vi "Init Error Logging.vi"(8 "error in (no error)":errorcluster, 11 "SOL-Server in":refnum<class "SOL-Server.lvclass">) -> (0 "error out":errorcluster, 3 "SOL-Server out":refnum<class "SOL-Server.lvclass">)   [LabVIEW 2020, in "Summer of LabVIEW.lvlib" / "SOL-Server.lvclass"]
uses:
  SOL-Server.lvclass
  SOL-Server.lvclass/SOL-Server.ctl
  Error Log.ctl
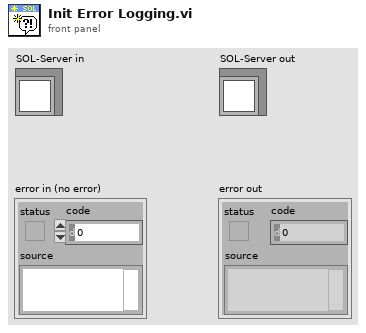
[diagram p1: front panel]
types:
  T1 = typedef "Summer of LabVIEW.lvlib/SOL-Server.lvclass/Error Log.ctl" = cluster{"Time Stamp":timestamp, "Code":i32, "Source":string}
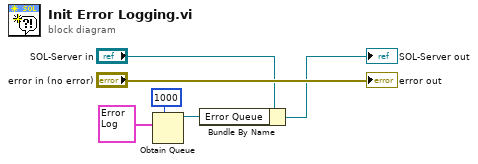
[diagram p0: block diagram]
diagram:
  n1 = Obtain Queue(max queue size (-1, unlimited)=1000, element data type=T1 {"Time Stamp"=timestamp(0 s since 1904-01-01), "Code"=0, "Source"=""} ("Error Log")) -> (queue out=w1:refnum<queue>)  [unwired: 3 in, 2 out]
  n2 = Bundle By Name(cluster="SOL-Server in", "Error Queue"=w1) -> (→"SOL-Server out":refnum<class "SOL-Server.lvclass">)
  "error out" <- "error in (no error)"
